vi "Read BG Loops.vi"(8 "error in (no error)":errorcluster, 11 "Worker Actor in":refnum<class "Worker Actor.lvclass">) -> (0 "error out":errorcluster, 2 "BG Loops":set{i32}(c389), 3 "Worker Actor out":refnum<class "Worker Actor.lvclass">)   [LabVIEW 2021, in "Worker Actor.lvclass"]
uses:
  Worker Actor.lvclass
  Worker Actor.lvclass/Worker Actor.ctl
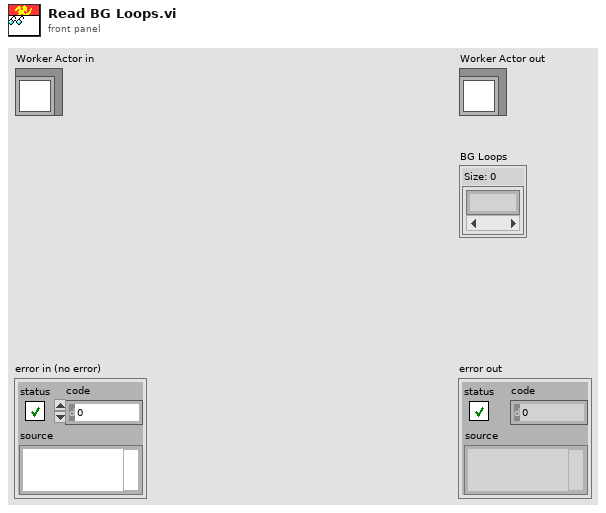
[diagram p1: front panel]
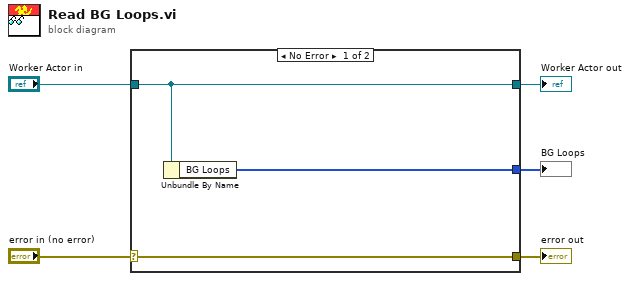
[diagram p0: block diagram]
diagram:
  n1 = case shown="No Error" "error in (no error)" {
    selector: "error in (no error)" -> [w8 w9]
    tunnel: [w8 w9] -> w4
    tunnel: [w7 w10] -> w2
    tunnel: "Worker Actor in" -> [w7 w10]
    tunnel: [w6 _] -> w1
    frame No Error {
      n2 = Unbundle By Name(w7) -> ("BG Loops"=w6:i32[])
    }
    frame Error {
    }
  }
  "error out" <- w4
  "Worker Actor out" <- w2
  "BG Loops" <- w1
